vi "Read All Tables.vi"(1 "Error In":errorcluster) -> (0 "Error Out":errorcluster)   [LabVIEW 2018]
uses:
  Type Defs/State Machine.ctl
  Type Defs/Global Action.ctl
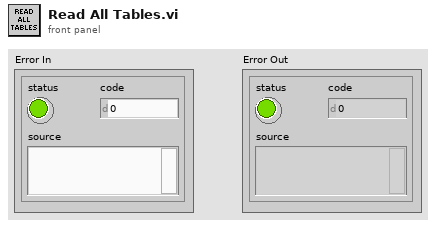
[diagram p1: front panel]
types:
  T1 = typedef "State Machine.ctl" = enum16{"Case 0", "Case 1", "Case 2", "Case 3", "Case 4", "Case 5", "Case 6", "Case 7", "Case 8", "Case 9", "Case 10", "Case 11", "Case 12", "Case 13", "Case 14", "Case 15", "Case 16", "Error", "Exit"}
  T2 = typedef "Global Action.ctl" = enum16{"Write", "Read"}
  T3 = typedef "CAL_RES.ctl" = cluster{"Calibrations":cluster{"Q1 +ve":dbl[][], "Q2 +ve":dbl[][], "Q1 -ve":dbl[][], "Q2 -ve":dbl[][]}, "Resolution Q1":cluster{"High +ve":dbl[][], "Med +ve":dbl[][], "Low +ve":dbl[][], "High -ve":dbl[][], "Med -ve":dbl[][], "Low -ve":dbl[][]}, "Resolution Q2":cluster{"High +ve":dbl[][], "Med +ve":dbl[][], "Low +ve":dbl[][], "High -ve":dbl[][], "Med -ve":dbl[][], "Low -ve":dbl[][]}}
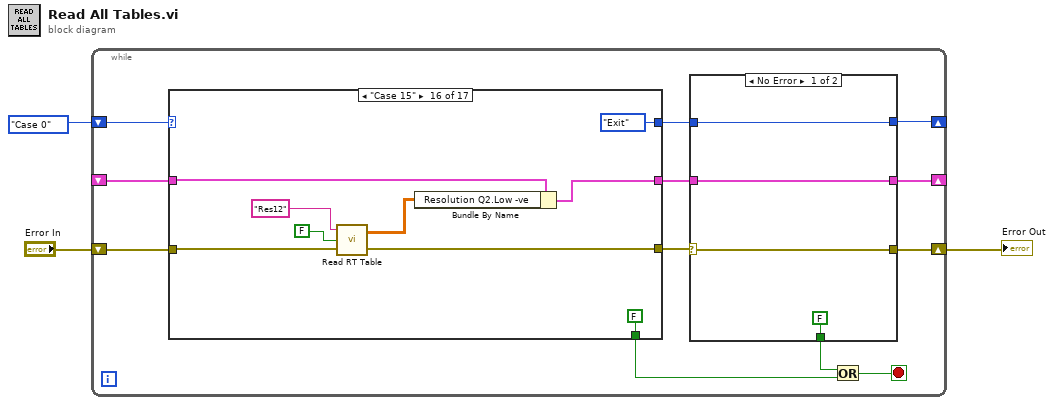
[diagram p0: block diagram]
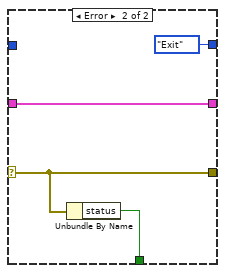
[diagram p2: hidden frame]
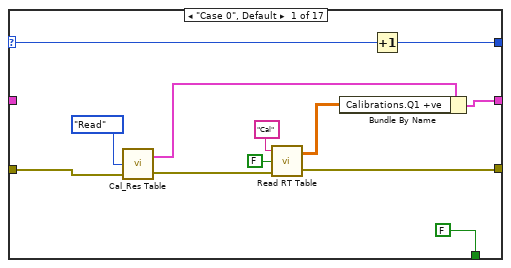
[diagram p3: hidden frame]
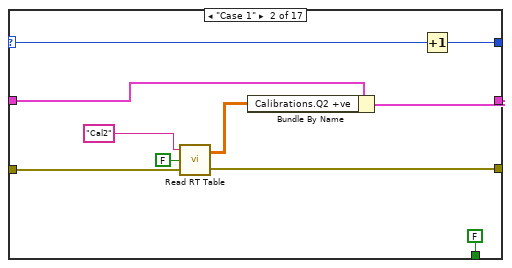
[diagram p4: hidden frame]
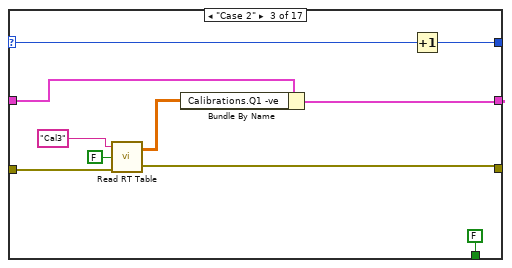
[diagram p5: hidden frame]
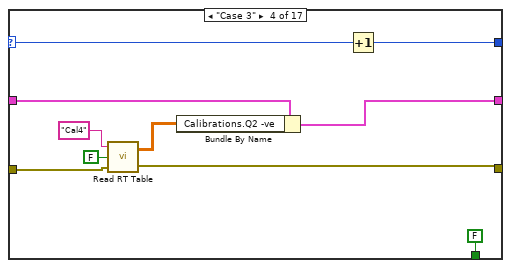
[diagram p6: hidden frame]
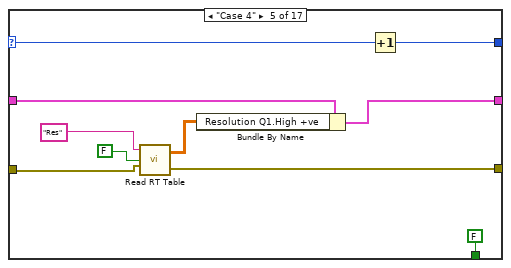
[diagram p7: hidden frame]
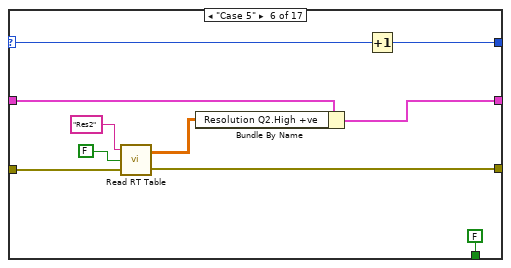
[diagram p8: hidden frame]
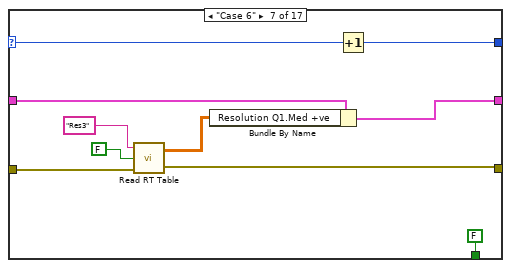
[diagram p9: hidden frame]
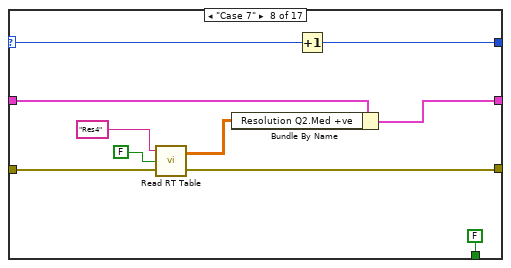
[diagram p10: hidden frame]
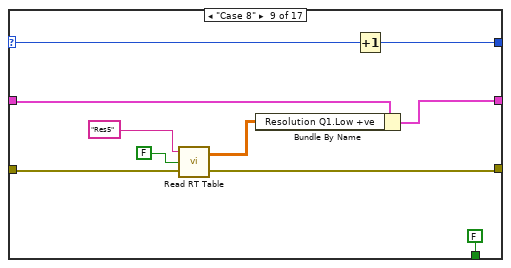
[diagram p11: hidden frame]
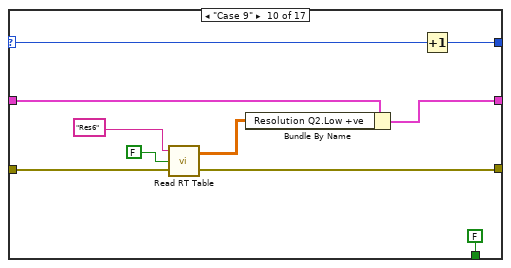
[diagram p12: hidden frame]
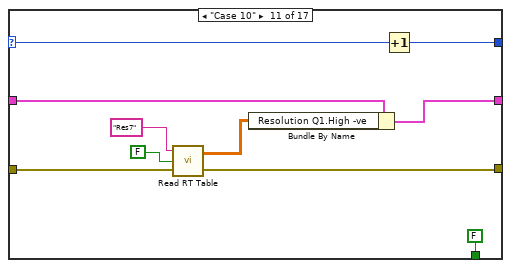
[diagram p13: hidden frame]
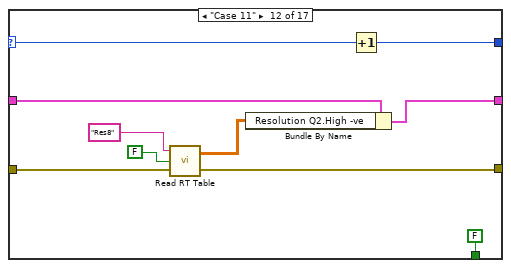
[diagram p14: hidden frame]
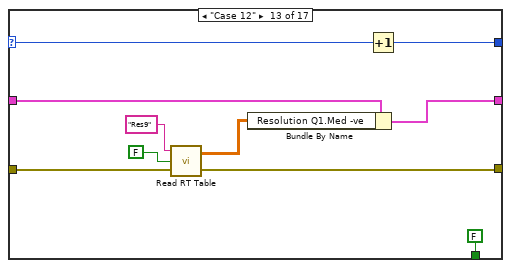
[diagram p15: hidden frame]
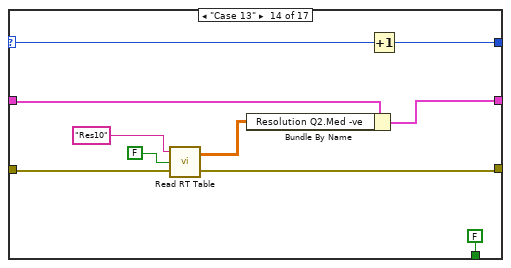
[diagram p16: hidden frame]
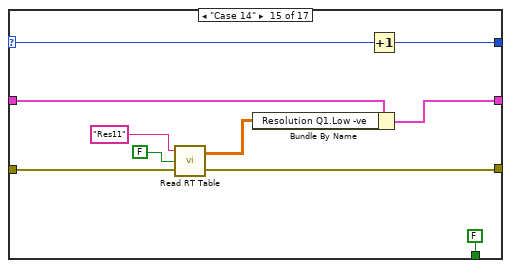
[diagram p17: hidden frame]
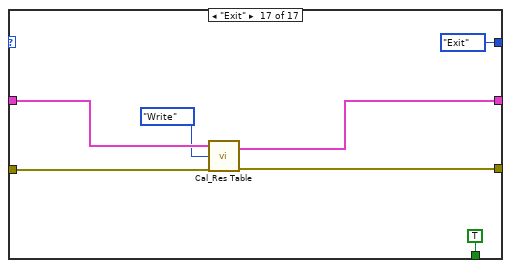
[diagram p18: hidden frame]
diagram:
  n1 = while {
    shift-right: [w12] -> w1
    shift-left: "Error In" -> [w14]
    shift-right: [w10] -> _
    shift-left: State_Machine."Case 0" ("Enum") -> [w15]
    shift-right: [w5] -> _
    shift-left: _ -> [w4]
    stop <- w9 stop-if-true
    n2 = case shown="\"Case 15\"" w15 {
      selector: w15 -> [w29 w45 w48 w57 w68 w82 w89 w99 w109 w119 w129 w139 w149 w158 w169 _ _]
      tunnel: w14 -> [w30 w43 w53 w61 w70 w84 w91 w103 w112 w121 w132 w143 w153 w163 w173 w181 w191]
      tunnel: [w25 w39 w47 w58 w71 w83 w90 w102 w111 w120 w131 w140 w151 w161 w170 w178 w188] -> w13
      tunnel: [w24 w36 w46 w56 w66 w76 w86 w96 w106 w116 w126 w136 w146 w156 w166 State_Machine."Exit" ("Enum") State_Machine."Exit" ("Enum")] -> w11
      tunnel: [FALSE FALSE FALSE FALSE FALSE FALSE FALSE FALSE FALSE FALSE FALSE FALSE FALSE FALSE FALSE FALSE TRUE] -> w7
      tunnel: [w26 w38 w51 w60 w72 w79 w93 w100 w110 w122 w130 w141 w150 w160 w171 w179 w189] -> w6
      tunnel: w4 -> [_ w42 w52 w62 w73 w80 w92 w101 w113 w123 w133 w142 w152 w162 w172 w180 w190]
      frame "Case 0", Default {
        n3 = call "Cal_Res Table.vi"("Error In"=w30, "Action"=Global_Action."Read") -> ("Error Out"=w33:errorcluster, "Parameters Out"=w31:T3)  [unwired: 1 in]
        n4 = call "Read RT Table.vi"("error in (no error)"=w33, "Simulator"=FALSE, "key"="Cal") -> ("error out"=w25:errorcluster, "Table"=w32:dbl[][])
        n5 = Bundle By Name(cluster=w31, "Calibrations.Q1 +ve"=w32) -> (w26:T3)
        n6 = Increment(x=w29) -> (x+1=w24:T1)
      }
      frame "Case 1" {
        n7 = call "Read RT Table.vi"("error in (no error)"=w43, "Simulator"=FALSE, "key"="Cal2") -> ("error out"=w39:errorcluster, "Table"=w44:dbl[][])
        n8 = Bundle By Name(cluster=w42, "Calibrations.Q2 +ve"=w44) -> (w38:T3)
        n9 = Increment(x=w45) -> (x+1=w36:T1)
      }
      frame "Case 2" {
        n10 = call "Read RT Table.vi"("error in (no error)"=w53, "Simulator"=FALSE, "key"="Cal3") -> ("error out"=w47:errorcluster, "Table"=w55:dbl[][])
        n11 = Bundle By Name(cluster=w52, "Calibrations.Q1 -ve"=w55) -> (w51:T3)
        n12 = Increment(x=w48) -> (x+1=w46:T1)
      }
      frame "Case 3" {
        n13 = call "Read RT Table.vi"("error in (no error)"=w61, "Simulator"=FALSE, "key"="Cal4") -> ("error out"=w58:errorcluster, "Table"=w65:dbl[][])
        n14 = Bundle By Name(cluster=w62, "Calibrations.Q2 -ve"=w65) -> (w60:T3)
        n15 = Increment(x=w57) -> (x+1=w56:T1)
      }
      frame "Case 4" {
        n16 = call "Read RT Table.vi"("error in (no error)"=w70, "Simulator"=FALSE, "key"="Res") -> ("error out"=w71:errorcluster, "Table"=w75:dbl[][])
        n17 = Bundle By Name(cluster=w73, "Resolution Q1.High +ve"=w75) -> (w72:T3)
        n18 = Increment(x=w68) -> (x+1=w66:T1)
      }
      frame "Case 5" {
        n19 = call "Read RT Table.vi"("error in (no error)"=w84, "Simulator"=FALSE, "key"="Res2") -> ("error out"=w83:errorcluster, "Table"=w78:dbl[][])
        n20 = Bundle By Name(cluster=w80, "Resolution Q2.High +ve"=w78) -> (w79:T3)
        n21 = Increment(x=w82) -> (x+1=w76:T1)
      }
      frame "Case 6" {
        n22 = call "Read RT Table.vi"("error in (no error)"=w91, "Simulator"=FALSE, "key"="Res3") -> ("error out"=w90:errorcluster, "Table"=w94:dbl[][])
        n23 = Bundle By Name(cluster=w92, "Resolution Q1.Med +ve"=w94) -> (w93:T3)
        n24 = Increment(x=w89) -> (x+1=w86:T1)
      }
      frame "Case 7" {
        n25 = call "Read RT Table.vi"("error in (no error)"=w103, "Simulator"=FALSE, "key"="Res4") -> ("error out"=w102:errorcluster, "Table"=w104:dbl[][])
        n26 = Bundle By Name(cluster=w101, "Resolution Q2.Med +ve"=w104) -> (w100:T3)
        n27 = Increment(x=w99) -> (x+1=w96:T1)
      }
      frame "Case 8" {
        n28 = call "Read RT Table.vi"("error in (no error)"=w112, "Simulator"=FALSE, "key"="Res5") -> ("error out"=w111:errorcluster, "Table"=w114:dbl[][])
        n29 = Bundle By Name(cluster=w113, "Resolution Q1.Low +ve"=w114) -> (w110:T3)
        n30 = Increment(x=w109) -> (x+1=w106:T1)
      }
      frame "Case 9" {
        n31 = call "Read RT Table.vi"("error in (no error)"=w121, "Simulator"=FALSE, "key"="Res6") -> ("error out"=w120:errorcluster, "Table"=w124:dbl[][])
        n32 = Bundle By Name(cluster=w123, "Resolution Q2.Low +ve"=w124) -> (w122:T3)
        n33 = Increment(x=w119) -> (x+1=w116:T1)
      }
      frame "Case 10" {
        n34 = call "Read RT Table.vi"("error in (no error)"=w132, "Simulator"=FALSE, "key"="Res7") -> ("error out"=w131:errorcluster, "Table"=w134:dbl[][])
        n35 = Bundle By Name(cluster=w133, "Resolution Q1.High -ve"=w134) -> (w130:T3)
        n36 = Increment(x=w129) -> (x+1=w126:T1)
      }
      frame "Case 11" {
        n37 = call "Read RT Table.vi"("error in (no error)"=w143, "Simulator"=FALSE, "key"="Res8") -> ("error out"=w140:errorcluster, "Table"=w144:dbl[][])
        n38 = Bundle By Name(cluster=w142, "Resolution Q2.High -ve"=w144) -> (w141:T3)
        n39 = Increment(x=w139) -> (x+1=w136:T1)
      }
      frame "Case 12" {
        n40 = call "Read RT Table.vi"("error in (no error)"=w153, "Simulator"=FALSE, "key"="Res9") -> ("error out"=w151:errorcluster, "Table"=w154:dbl[][])
        n41 = Bundle By Name(cluster=w152, "Resolution Q1.Med -ve"=w154) -> (w150:T3)
        n42 = Increment(x=w149) -> (x+1=w146:T1)
      }
      frame "Case 13" {
        n43 = call "Read RT Table.vi"("error in (no error)"=w163, "Simulator"=FALSE, "key"="Res10") -> ("error out"=w161:errorcluster, "Table"=w164:dbl[][])
        n44 = Bundle By Name(cluster=w162, "Resolution Q2.Med -ve"=w164) -> (w160:T3)
        n45 = Increment(x=w158) -> (x+1=w156:T1)
      }
      frame "Case 14" {
        n46 = call "Read RT Table.vi"("error in (no error)"=w173, "Simulator"=FALSE, "key"="Res11") -> ("error out"=w170:errorcluster, "Table"=w174:dbl[][])
        n47 = Bundle By Name(cluster=w172, "Resolution Q1.Low -ve"=w174) -> (w171:T3)
        n48 = Increment(x=w169) -> (x+1=w166:T1)
      }
      frame "Case 15" {
        n49 = call "Read RT Table.vi"("error in (no error)"=w181, "Simulator"=FALSE, "key"="Res12") -> ("error out"=w178:errorcluster, "Table"=w183:dbl[][])
        n50 = Bundle By Name(cluster=w180, "Resolution Q2.Low -ve"=w183) -> (w179:T3)
      }
      frame "Exit" {
        n51 = call "Cal_Res Table.vi"("Error In"=w191, "Action"=Global_Action."Write", "Parameters In"=w190) -> ("Error Out"=w188:errorcluster, "Parameters Out"=w189:T3)
      }
    }
    n52 = case shown="No Error" w13 {
      selector: w13 -> [w19 w21]
      tunnel: [w19 w21] -> w12
      tunnel: w11 -> [w16 _]
      tunnel: [w16 State_Machine."Exit"] -> w10
      tunnel: [FALSE ("status") w22] -> w8
      tunnel: w6 -> [w17 w20]
      tunnel: [w17 w20] -> w5
      frame No Error {
      }
      frame Error {
        n53 = Unbundle By Name(w21) -> ("status"=w22:bool)
      }
    }
    n54 = Or(x=w8, y=w7) -> (x .or. y?=w9:bool)
  }
  "Error Out" <- w1
